vi "GetMeasBands.vi"(6 "Legacy (f)?":bool, 8 "error in (no error)":errorcluster) -> (0 "error out":errorcluster, 2 "TestSet Models":string[](array[string]), 3 "TestSets":T1[](array[typedef]))   [LabVIEW 2011]
uses:
  Test Set Definition.ctl
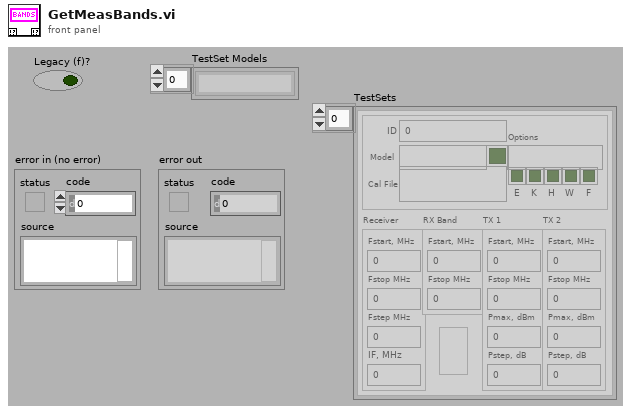
[diagram p1: front panel]
types:
  T1 = typedef "Test Set Definition.ctl" = cluster{"General":cluster{"ID":u32, "Model":string, "Dual Port?":bool, "Options":string, "Options":cluster{"E":bool, "K":bool, "H":bool, "W":bool, "F":bool}, "Cal File":path}, "Receiver":cluster{"Fstart, MHz":dbl, "Fstop MHz":dbl, "Fstep MHz":dbl, "IF, MHz":dbl}, "RX Band":cluster{"Fstart, MHz":dbl, "Fstop MHz":dbl}, "TX 1":cluster{"Fstart, MHz":dbl, "Fstop MHz":dbl, "Pmax, dBm":dbl, "Pstep, dB":dbl}, "TX 2":cluster{"Fstart, MHz":dbl, "Fstop MHz":dbl, "Pmax, dBm":dbl, "Pstep, dB":dbl}, "Low-side?":bool}
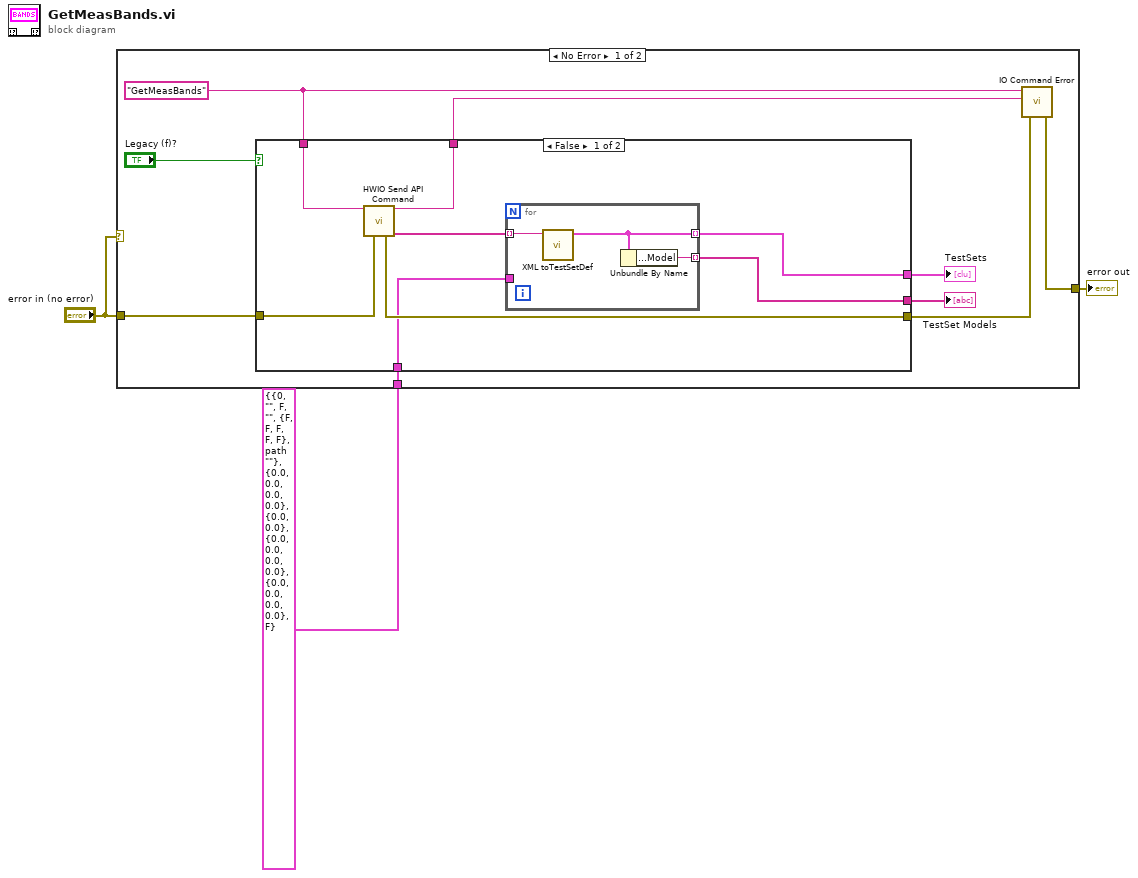
[diagram p0: block diagram]
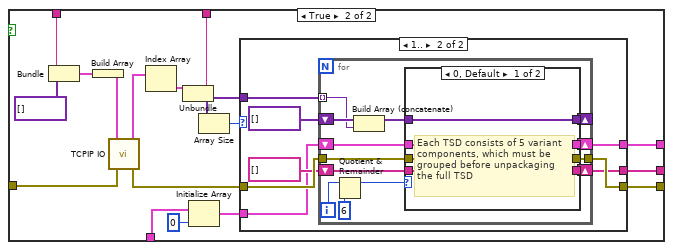
[diagram p2: hidden frame]
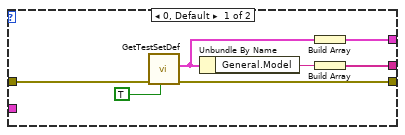
[diagram p3: hidden frame]
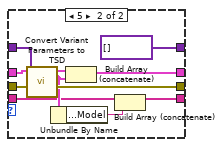
[diagram p4: hidden frame]
diagram:
  n1 = case shown="No Error" "error in (no error)" {
    tunnel: "error in (no error)" -> [w12 w83]
    tunnel: [w10 w83] -> w3
    tunnel: T1 {"General"={"ID"=0, "Model"="", "Dual Port?"=FALSE, "Options"="", "Options"={"E"=FALSE, "K"=FALSE, "H"=FALSE, "W"=FALSE, "F"=FALSE}, "Cal File"=path ""}, "Receiver"={"Fstart, MHz"=0.0, "Fstop MHz"=0.0, "Fstep MHz"=0.0, "IF, MHz"=0.0}, "RX Band"={"Fstart, MHz"=0.0, "Fstop MHz"=0.0}, "TX 1"={"Fstart, MHz"=0.0, "Fstop MHz"=0.0, "Pmax, dBm"=0.0, "Pstep, dB"=0.0}, "TX 2"={"Fstart, MHz"=0.0, "Fstop MHz"=0.0, "Pmax, dBm"=0.0, "Pstep, dB"=0.0}, "Low-side?"=FALSE} ("TestSetDef") -> [w7 _]
    frame No Error {
      w8 = "GetMeasBands"
      n2 = case shown="False" "Legacy (f)?" {
        tunnel: w12 -> [w18 w39]
        tunnel: [w17 w37] -> w11
        tunnel: [w19 w36] -> w9
        tunnel: w8 -> [w20 w35]
        tunnel: w7 -> [w15 w28]
        tunnel: [w14 w30] -> w6
        tunnel: [w13 w29] -> w5
        frame False {
          n3 = call "HWIO Send API Command.vi"("Action"=w20, "error in (no error)"=w18) -> ("Action out"=w19:string, "error out"=w17:errorcluster, "String out"=w16:string[])  [unwired: 6 in, 5 out]
          n4 = for {
            tunnel: w16 -> [w22] mode=indexing
            tunnel: w15 -> [_]
            tunnel: [w21] -> w14 mode=indexing
            tunnel: [w23] -> w13 mode=indexing
            n5 = call "XML toTestSetDef.vi"("TSD XML"=w22) -> ("Test Set Definition"=w21:T1)  [unwired: 10 in]
            n6 = Unbundle By Name(w21) -> ("General.Model"=w23:string)
          }
        }
        frame True {
          n7 = Bundle(w35, "appended array"=variant[] []) -> (w40:cluster{string, "appended array":variant[]})  [unwired: 1 out]
          n8 = Build Array(w40) -> (w32:cluster{string, "appended array":variant[]}[])
          n9 = call "TCPIP IO.vi"("error in (no error)"=w39, "Commands"=w32) -> ("error out"=w38:errorcluster, "Responses"=w34:cluster{string, variant[]}[])  [unwired: 1 in, 3 out]
          n10 = Index Array(array=w34) -> (element=w33:cluster{string, variant[]})  [unwired: 1 in]
          n11 = Unbundle(w33) -> (w36:string, w25:variant[])
          n12 = Initialize Array(w28, 0 ("dimension size")) -> (w26:T1[])
          n13 = Array Size(array=w25) -> (size(s)=w24:i32)
          n14 = case shown="1.." w24 {
            tunnel: w38 -> [w47 w55]
            tunnel: [w45 w54] -> w37
            tunnel: [w42 w52] -> w30
            tunnel: [w44 w50] -> w29
            tunnel: w26 -> [_ w49]
            tunnel: w25 -> [_ w48]
            frame 0, Default {
              n15 = call "GetTestSetDef.vi"("Legacy (f)?"=TRUE, "error in (no error)"=w47) -> ("error out"=w45:errorcluster, "TestSetDef"=w41:T1)  [unwired: 8 in]
              n16 = Unbundle By Name(w41) -> ("General.Model"=w43:string)
              n17 = Build Array(w41) -> (w42:T1[])
              n18 = Build Array(w43) -> (w44:string[])
            }
            frame 1.. {
              n19 = for {
                tunnel: [w58] -> w54
                tunnel: w55 -> [w61]
                tunnel: w48 -> [w64] mode=indexing
                shift-right: [w62] -> _
                shift-left: variant[] [] -> [w65]
                shift-right: [w60] -> w52
                shift-left: w49 -> [w59]
                shift-right: [w56] -> w50
                shift-left: string[] [] ("TestSet Models") -> [w57]
                i -> [w68]
                n20 = Quotient & Remainder(x=w68, y=6) -> (x-y*floor(x/y)=w66:i32)  [unwired: 1 out]
                n21 = Build Array (concatenate)(w65, w64) -> (w63:variant[])
                n22 = case shown="0, Default" w66 {
                  tunnel: w63 -> [w72 w82]
                  tunnel: [w72 variant[] []] -> w62
                  tunnel: w61 -> [w71 w81]
                  tunnel: [w70 w80] -> w60
                  tunnel: w59 -> [w70 w77]
                  tunnel: [w71 w79] -> w58
                  tunnel: w57 -> [w69 w75]
                  tunnel: [w69 w73] -> w56
                  frame 0, Default {
                    # "Each TSD consists of 5 variant\ncomponents, which must be\ngrouped before unpackaging\nthe full TSD"
                  }
                  frame 5 {
                    n23 = call "Convert Variant Parameters to TSD.vi"("error in"=w81, "Variant Parameter Array"=w82) -> ("error out"=w79:errorcluster, "TestSetDef"=w76:T1)  [unwired: 8 out]
                    n24 = Unbundle By Name(w76) -> ("General.Model"=w74:string)
                    n25 = Build Array (concatenate)(w77, w76) -> (w80:T1[])
                    n26 = Build Array (concatenate)(w75, w74) -> (w73:string[])
                  }
                }
              }
            }
          }
        }
      }
      "TestSets" <- w6
      "TestSet Models" <- w5
      n27 = call "IO Command Error.vi"("error in (no error)"=w11, "Command Returned (\"\")"=w9, "Command Sent (\"\")"=w8) -> ("error out"=w10:errorcluster)  [unwired: 4 out]
    }
    frame Error {
    }
  }
  "error out" <- w3
